vi "Read Header.vi"(8 "error in (no error)":errorcluster, 11 "Logs in":refnum<class "Logs.lvclass">) -> (0 "error out":errorcluster, 2 "Header":string[](array[string]), 3 "Logs out":refnum<class "Logs.lvclass">)   [LabVIEW 2019, in "Logs.lvclass"]
uses:
  Logs.lvclass
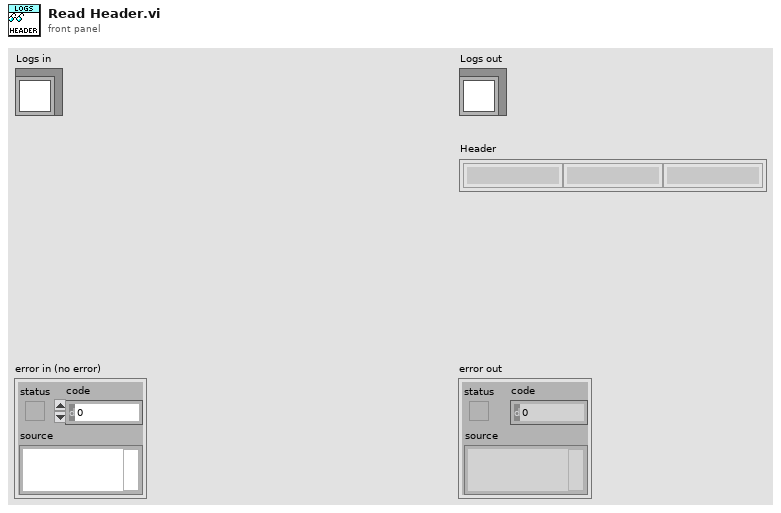
[diagram p1: front panel]
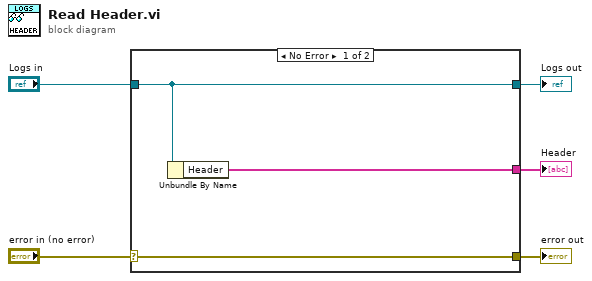
[diagram p0: block diagram]
diagram:
  n1 = case shown="No Error" "error in (no error)" {
    selector: "error in (no error)" -> [w8 w9]
    tunnel: [w8 w9] -> w4
    tunnel: [w7 w10] -> w2
    tunnel: "Logs in" -> [w7 w10]
    tunnel: [w6 _] -> w1
    frame No Error {
      n2 = Unbundle By Name(w7) -> ("Header"=w6:string[])
    }
    frame Error {
    }
  }
  "error out" <- w4
  "Logs out" <- w2
  "Header" <- w1
